vi "ElevShiftStatus.vi"(10 "Update?":bool, 11 "ElevShiftStatusIn":bool) -> (3 "ElevShiftStatusOut":bool)   [LabVIEW 2017]
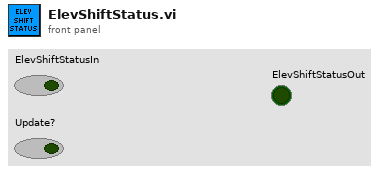
[diagram p1: front panel]
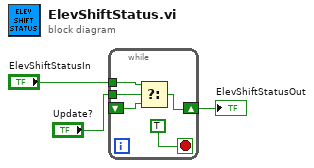
[diagram p0: block diagram]
diagram:
  n1 = while {
    tunnel: "Update?" -> [w8]
    tunnel: "ElevShiftStatusIn" -> [w7]
    shift-right: [w6] -> w1
    shift-left: _ -> [w5]
    stop <- TRUE stop-if-true
    n2 = Select(t=w7, s=w8, f=w5) -> (s? t:f=w6:bool)
  }
  "ElevShiftStatusOut" <- w1
